vi "1.2 数据操作时间字符串.vi"() -> ()   [LabVIEW 2022 SP3]
panel:
  out "输出 1":timestamp
  out "双精度浮点数":dbl
  out "日期/时间字符串":string
  out "当前时间":timestamp
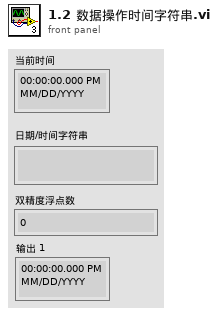
[diagram p1: front panel]
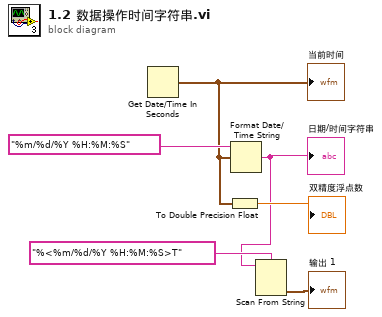
[diagram p0: block diagram]
diagram:
  n1 = Get Date/Time In Seconds() -> (seconds since 1Jan1904=w5:timestamp)
  "当前时间" <- w5
  n2 = To Double Precision Float(number=w5) -> (double precision float=→"双精度浮点数":dbl)
  n3 = Format Date/Time String ("格式化日期/时间字符串")(time format string (%c)="%m/%d/%Y %H:%M:%S" ("日期/时间字符串"), seconds (now)=w5) -> (date/time string=w2:string)  [unwired: 1 in]
  "日期/时间字符串" <- w2
  n4 = Scan From String(format string="%<%m/%d/%Y %H:%M:%S>T" ("日期/时间字符串"), input string=w2) -> (output 1=→"输出 1":timestamp)  [unwired: 3 in, 3 out]
